vi "Semaphore to eliminate race condition.vi"() -> ()   [LabVIEW 2012]
panel:
  out "Loop 2":i32
  out "Loop 1":i32
  in  "stop 2":bool
  in  "stop":bool
  in  "Input":dbl
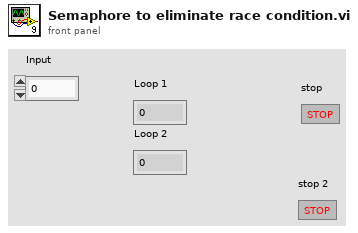
[diagram p1: front panel]
types:
  T1 = typedef "Semaphore RefNum" = refnum<k1>
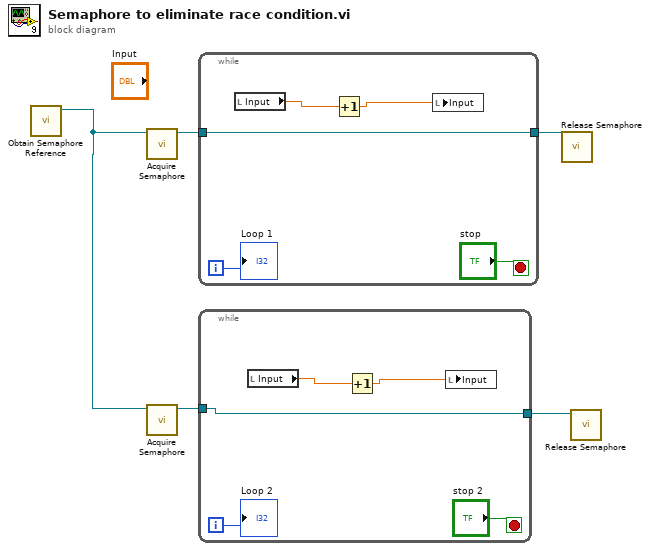
[diagram p0: block diagram]
diagram:
  n1 = call <vilib>:"Obtain Semaphore Reference.vi"() -> ("semaphore"=w5:T1)  [unwired: 5 in, 2 out]
  n2 = call <vilib>:"Acquire Semaphore.vi"("semaphore"=w5) -> ("semaphore out"=w4:T1)  [unwired: 4 in, 2 out]
  n3 = call <vilib>:"Acquire Semaphore.vi"("semaphore"=w5) -> ("semaphore out"=w3:T1)  [unwired: 4 in, 2 out]
  n4 = while {
    tunnel: w4 -> [w7]
    tunnel: [w7] -> w2
    i -> [w6]
    stop <- "stop" stop-if-true
    n5 = local read "Input"() -> (w10:dbl)
    n6 = Increment(x=w10) -> (x+1=w9:dbl)
    n7 = local write "Input"(w9) -> ()
    "Loop 1" <- w6
  }
  n8 = while {
    tunnel: w3 -> [w12]
    tunnel: [w12] -> w1
    i -> [w11]
    stop <- "stop 2" stop-if-true
    n9 = local read "Input"() -> (w14:dbl)
    n10 = Increment(x=w14) -> (x+1=w15:dbl)
    n11 = local write "Input"(w15) -> ()
    "Loop 2" <- w11
  }
  n12 = call <vilib>:"Release Semaphore.vi"("semaphore"=w2) -> ()  [unwired: 5 in, 2 out]
  n13 = call <vilib>:"Release Semaphore.vi"("semaphore"=w1) -> ()  [unwired: 5 in, 2 out]
